vi "CloseApp.vi"(2 "Error In":errorcluster, 3 "Show Front Panel?":bool) -> ()   [LabVIEW 2019]
panel:
  out "Time to close":dbl caption="Time to close application" format="%.1f s"
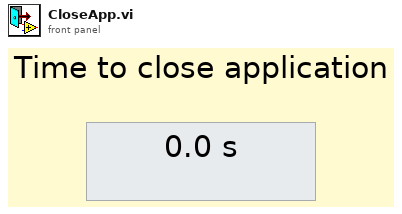
[diagram p1: front panel]
types:
  T1 = enum32{"Invalid", "Standard", "Closed", "Hidden", "Minimized", "Maximized"}
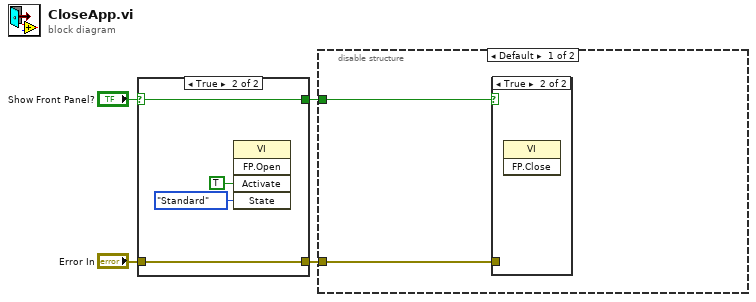
[diagram p0: block diagram]
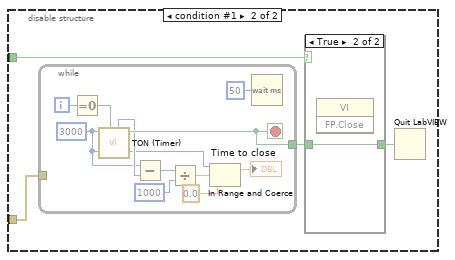
[diagram p3: hidden frame]
diagram:
  n1 = case shown="True" "Show Front Panel?" {
    selector: "Show Front Panel?" -> [w5 w7]
    tunnel: "Error In" -> [w6 w10]
    tunnel: [w6 w10] -> w3
    tunnel: [w5 w7] -> w1
    frame False {
    }
    frame True {
      n2 = invoke class="VI" method="FP.Open"("Activate"=TRUE ("Activate?"), "State"=T1."Standard") -> ()  [unwired: 3 in, 5 out]
    }
  }
  n3 = disable-structure shown="Default" {
    disable-tunnel: w3 -> [w11 w15]
    disable-tunnel: w1 -> [w12 w16]
    frame condition #0 (active) {
      n4 = case shown="True" w12 {
        tunnel: w11 -> [_ _]
        frame False {
        }
        frame True {
          n5 = invoke class="VI" method="FP.Close"() -> ()  [unwired: 3 in, 3 out]
        }
      }
    }
    frame condition #1 {
      n6 = while {
        tunnel: [w25] -> w14
        tunnel: w15 -> [_]
        i -> [w28]
        stop <- w25 stop-if-true
        w19 = u32 3000 ("Set Time")
        n7 = Equal To 0?(x=w28) -> (x = 0?=w27:bool)
        n8 = call "TON (Timer).vi"("Reset"=w27, "Set Time"=w19) -> ("Timeout"=w25:bool, "Elapsed Time"=w24:u32)  [unwired: 7 in, 1 out]
        n9 = Subtract(x=w19, y=w24) -> (x-y=w23:u32)
        n10 = Divide(x=w23, y=u32 1000) -> (x/y=w21:dbl)
        n11 = In Range and Coerce(upper limit=w19, x=w21, lower limit=0.0) -> (coerced(x)=→"Time to close":dbl)  [unwired: 1 out]
        n12 = Wait (ms)(milliseconds to wait=u32 50) -> ()  [unwired: 1 out]
      }
      n13 = case shown="True" w16 {
        tunnel: w14 -> [_ w17]
        tunnel: [_ w17] -> w13
        frame False {
        }
        frame True {
          n14 = invoke class="VI" method="FP.Close"() -> ()  [unwired: 3 in, 3 out]
        }
      }
      n15 = Quit LabVIEW(quit? (T)=w13) -> ()
    }
  }
